vi "GIMBALE (SubVI).vi"(8 "error In":errorcluster, 10 "GIMBALE Queue":refnum<queue>, 11 "Refnum in":refnum<k20>) -> ()   [LabVIEW 2015]
uses:
  PC/QMH Fundamentals - Message Cluster.ctl
  <vilib>/Utility/error.llb/Error Cluster From Error Code.vi
  <vilib>/rvi/errors/niLvFpgaAdjustHostInterfaceError.vi
  <vilib>/rvi/interface/nirviReadWriteControl/nirviReadWriteControl.xnode
  NiFpgaLv.dll
  <vilib>/rvi/interface/Simulation/niFpgaSimulationCallBeginRW.vi
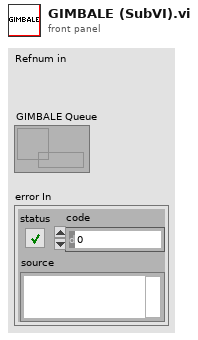
[diagram p1: front panel]
types:
  T1 = cluster{"bool":bool, "Gimbale":cluster{"PITCH 1":dbl, "YAW 1":dbl, "ROLL 1":dbl}}
  T2 = typedef "QMH Fundamentals - Message Cluster.ctl" = cluster{"Message":string, "Message Data":variant}
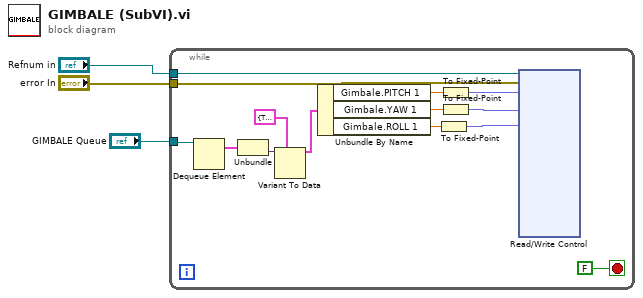
[diagram p0: block diagram]
diagram:
  n1 = while {
    tunnel: "error In" -> [w15]
    tunnel: "Refnum in" -> [w16]
    tunnel: "GIMBALE Queue" -> [w14]
    stop <- FALSE stop-if-true
    n2 = Dequeue Element(queue=w14) -> (element=w13:T2)  [unwired: 2 in, 3 out]
    n3 = Unbundle(w13) -> ("Message Data"=w12:variant)  [unwired: 1 out]
    n4 = Variant To Data(type=T1 {"bool"=TRUE, "Gimbale"={"PITCH 1"=0.0, "YAW 1"=0.0, "ROLL 1"=0.0}} ("jazda"), Variant=w12) -> (data=w11:T1)  [unwired: 1 in, 1 out]
    n5 = Unbundle By Name(w11) -> ("Gimbale.PITCH 1"=w10:dbl, "Gimbale.YAW 1"=w8:dbl, "Gimbale.ROLL 1"=w7:dbl)
    n6 = To Fixed-Point(number=w7) -> (fixed-point=w5:fxp<+,32,0>)  [unwired: 1 in]
    n7 = To Fixed-Point(number=w10) -> (fixed-point=w9:fxp<+,32,0>)  [unwired: 1 in]
    n8 = To Fixed-Point(number=w8) -> (fixed-point=w6:fxp<+,32,0>)  [unwired: 1 in]
    n9 = xnode "Read/Write Control"("FPGA VI Reference In"=w16, "error in"=w15, "PITCH 1"=w9, "ROLL1"=w6, "YAW1"=w5) -> ()  [unwired: 7 in, 2 out]
  }
